vi "Set wavegen SINe signal parameters.vi"(8 "error in (no error)":errorcluster {"code" format="%.0x"}, 9 "Wavegen parameters in":T2={"Frequency (Hz)"=1000.0, "Amplitude (V)"=1.0, "Offset (V)"=0.0, "Load Impedance"=enum."ONEMeg"} {"Offset (V)" format="%#_13g"; "Amplitude (V)" format="%#_13g"; "Frequency (Hz)" min=0.1 max=20000000.0 format="%#_13g"}, 11 "instrument handle in":refnum<k15>) -> (0 "error out":errorcluster, 2 "log string out":string, 3 "instrument handle out":refnum<k15>)   [LabVIEW 2017]
uses:
  Load Impedance.ctl
  Waveform type.ctl
  <instrlib>/Keysight InfiniiVision/Keysight InfiniiVision.lvlib
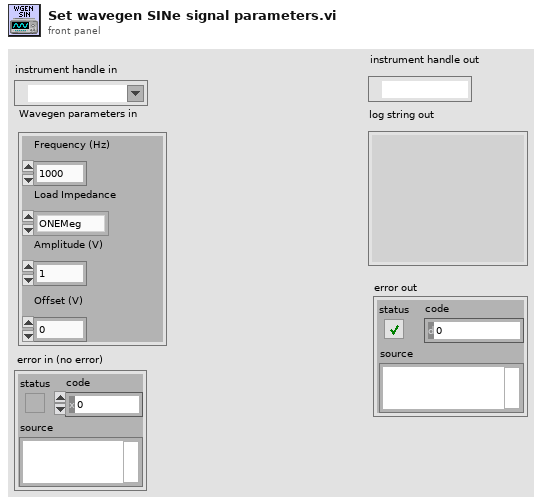
[diagram p1: front panel]
types:
  T1 = typedef "Load Impedance.ctl" = enum16{"ONEMeg", "FIFTy"}
  T2 = cluster{"Frequency (Hz)":dbl, "Amplitude (V)":dbl, "Offset (V)":dbl, "Load Impedance":T1}
  T3 = typedef "Waveform type.ctl" = enum16{"SINe", "SQUare", "RAMP", "PULSe", "DC", "NOISe"}
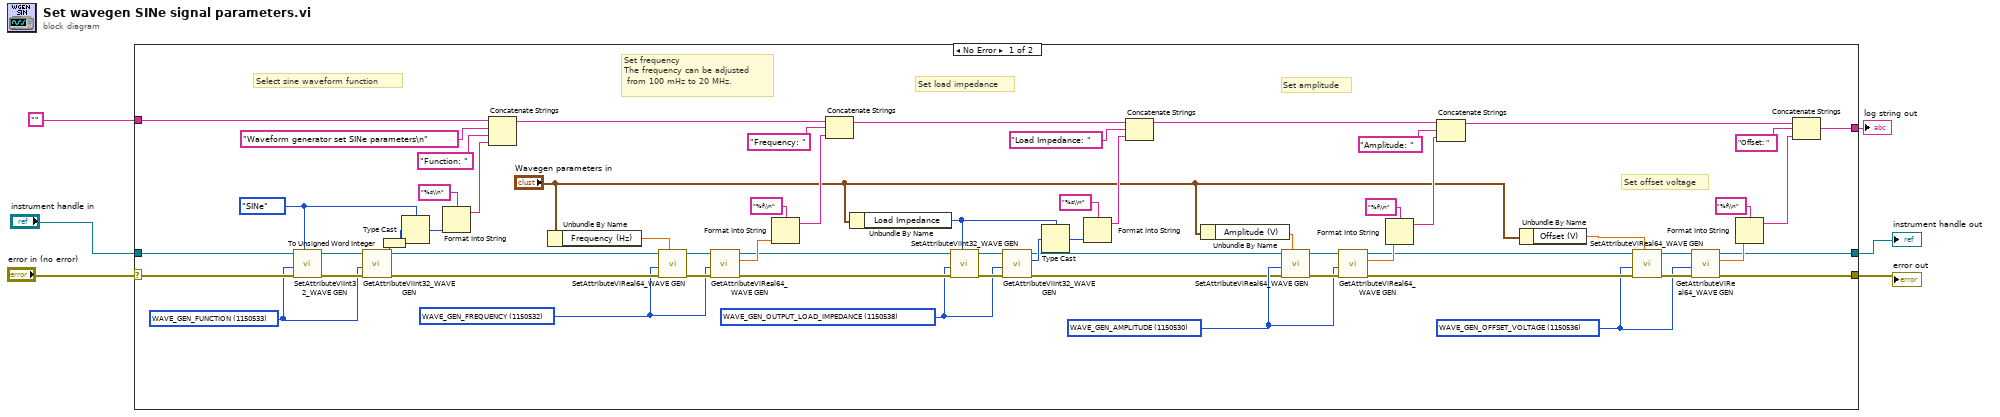
[diagram p0: block diagram]
diagram:
  n1 = case shown="No Error" "error in (no error)" {
    selector: "error in (no error)" -> [w68 w70]
    tunnel: "instrument handle in" -> [w69 w71]
    tunnel: [w34 w71] -> w2
    tunnel: [w33 w70] -> w1
    tunnel: [w32 w72] -> w3
    tunnel: "" ("log string in") -> [w30 w72]
    frame No Error {
      w22 = u32 1150538 items=["ARBITRARY_BYTE_ORDER"=1150415, "MODULATION_FUNCTION"=1150552, "MODULATION_TYPE"=1150555, "TRACKING_PHASE"=1150659, "WAVE_GEN_ADDITIONAL_NOISE"=1150529, "WAVE_GEN_ARBITRARY_BYTE_ORDER"=1150544, "WAVE_GEN_FUNCTION"=1150533, "WAVE_GEN_OUTPUT_LOAD_IMPEDANCE"=1150538, "WAVE_GEN_OUTPUT_MODE"=1150658] ("AttributeID")
      w27 = u32 1150536 items=["FM_DEVIATION"=1150548, "FM_FREQUENCY"=1150549, "FSK_FREQUENCY"=1150550, "FSK_MODULATION_RATE"=1150551, "MODULATION_RAMP_SYMMETRY"=1150553, "WAVE_GEN_AM_DEPTH"=1150546, "WAVE_GEN_AM_FREQUENCY"=1150547, "WAVE_GEN_AMPLITUDE"=1150530, "WAVE_GEN_DUTY_CYCLE"=1150531, "WAVE_GEN_FREQUENCY"=1150532, "WAVE_GEN_HIGH_VOLTAGE"=1150534, "WAVE_GEN_LOW_VOLTAGE"=1150535, "WAVE_GEN_OFFSET_VOLTAGE"=1150536, "WAVE_GEN_PERIOD"=1150539, "WAVE_GEN_PULSE_WIDTH"=1150540, "WAVE_GEN_RAMP_SYMMETRY"=1150541] ("AttributeID")
      w57 = Waveform_type."SINe"
      w28 = u32 1150530 items=["FM_DEVIATION"=1150548, "FM_FREQUENCY"=1150549, "FSK_FREQUENCY"=1150550, "FSK_MODULATION_RATE"=1150551, "MODULATION_RAMP_SYMMETRY"=1150553, "WAVE_GEN_AM_DEPTH"=1150546, "WAVE_GEN_AM_FREQUENCY"=1150547, "WAVE_GEN_AMPLITUDE"=1150530, "WAVE_GEN_DUTY_CYCLE"=1150531, "WAVE_GEN_FREQUENCY"=1150532, "WAVE_GEN_HIGH_VOLTAGE"=1150534, "WAVE_GEN_LOW_VOLTAGE"=1150535, "WAVE_GEN_OFFSET_VOLTAGE"=1150536, "WAVE_GEN_PERIOD"=1150539, "WAVE_GEN_PULSE_WIDTH"=1150540, "WAVE_GEN_RAMP_SYMMETRY"=1150541] ("AttributeID")
      w29 = u32 1150532 items=["FM_DEVIATION"=1150548, "FM_FREQUENCY"=1150549, "FSK_FREQUENCY"=1150550, "FSK_MODULATION_RATE"=1150551, "MODULATION_RAMP_SYMMETRY"=1150553, "WAVE_GEN_AM_DEPTH"=1150546, "WAVE_GEN_AM_FREQUENCY"=1150547, "WAVE_GEN_AMPLITUDE"=1150530, "WAVE_GEN_DUTY_CYCLE"=1150531, "WAVE_GEN_FREQUENCY"=1150532, "WAVE_GEN_HIGH_VOLTAGE"=1150534, "WAVE_GEN_LOW_VOLTAGE"=1150535, "WAVE_GEN_OFFSET_VOLTAGE"=1150536, "WAVE_GEN_PERIOD"=1150539, "WAVE_GEN_PULSE_WIDTH"=1150540, "WAVE_GEN_RAMP_SYMMETRY"=1150541] ("AttributeID")
      w65 = u32 1150533 items=["ARBITRARY_BYTE_ORDER"=1150415, "MODULATION_FUNCTION"=1150552, "MODULATION_TYPE"=1150555, "TRACKING_PHASE"=1150659, "WAVE_GEN_ADDITIONAL_NOISE"=1150529, "WAVE_GEN_ARBITRARY_BYTE_ORDER"=1150544, "WAVE_GEN_FUNCTION"=1150533, "WAVE_GEN_OUTPUT_LOAD_IMPEDANCE"=1150538, "WAVE_GEN_OUTPUT_MODE"=1150658] ("AttributeID")
      # "Set load impedance"
      # "Set offset voltage"
      # "Set amplitude"
      # "Set frequency\nThe frequency can be adjusted\n from 100 mHz to 20 MHz."
      # "Select sine waveform function"
      n2 = call <instrlib>:"SetAttributeViInt32_WAVE GEN.vi"("AttributeValue"=w57, "error in (no error)"=w68, "AttributeID"=w65, "instrument handle"=w69) -> ("error out"=w66:errorcluster, "instrument handle out"=w67:refnum<k15>)  [unwired: 6 in]
      n3 = call <instrlib>:"GetAttributeViInt32_WAVE GEN.vi"("error in (no error)"=w66, "AttributeID"=w65, "instrument handle"=w67) -> ("error out"=w61:errorcluster, "AttributeValue"=w58:i32, "instrument handle out"=w62:refnum<k15>)  [unwired: 6 in]
      n4 = To Unsigned Word Integer(number=w58) -> (unsigned 16bit integer=w7:u16)
      n5 = Type Cast(type=w57, x=w7) -> (*(type *) &x=w56:T3)
      n6 = Format Into String(format string="%s\\n", w56) -> (resulting string=w55:string)  [unwired: 2 in, 1 out]
      n7 = Concatenate Strings(w30, "Waveform generator set SINe parameters\n" ("string"), "Function: " ("string"), w55) -> (w51:string)
      n8 = Unbundle By Name("Wavegen parameters in") -> ("Frequency (Hz)"=w12:dbl)
      n9 = call <instrlib>:"SetAttributeViReal64_WAVE GEN.vi"("AttributeValue"=w12, "error in (no error)"=w61, "AttributeID"=w29, "instrument handle"=w62) -> ("error out"=w63:errorcluster, "instrument handle out"=w64:refnum<k15>)  [unwired: 6 in]
      n10 = call <instrlib>:"GetAttributeViReal64_WAVE GEN.vi"("error in (no error)"=w63, "AttributeID"=w29, "instrument handle"=w64) -> ("error out"=w23:errorcluster, "AttributeValue"=w54:dbl, "instrument handle out"=w24:refnum<k15>)  [unwired: 6 in]
      n11 = Format Into String(format string="%f\\n", w54) -> (resulting string=w49:string)  [unwired: 2 in, 1 out]
      n12 = Concatenate Strings(w51, "Frequency: " ("string"), w49) -> (w17:string)
      n13 = Unbundle By Name("Wavegen parameters in") -> ("Load Impedance"=w11:T1)
      n14 = call <instrlib>:"SetAttributeViInt32_WAVE GEN.vi"("AttributeValue"=w11, "error in (no error)"=w23, "AttributeID"=w22, "instrument handle"=w24) -> ("error out"=w26:errorcluster, "instrument handle out"=w25:refnum<k15>)  [unwired: 6 in]
      n15 = call <instrlib>:"GetAttributeViInt32_WAVE GEN.vi"("error in (no error)"=w26, "AttributeID"=w22, "instrument handle"=w25) -> ("error out"=w14:errorcluster, "AttributeValue"=w19:i32, "instrument handle out"=w13:refnum<k15>)  [unwired: 6 in]
      n16 = Type Cast(type=w11, x=w19) -> (*(type *) &x=w21:T1)
      n17 = Format Into String(format string="%s\\n", w21) -> (resulting string=w16:string)  [unwired: 2 in, 1 out]
      n18 = Concatenate Strings(w17, "Load Impedance: " ("string"), w16) -> (w15:string)
      n19 = Unbundle By Name("Wavegen parameters in") -> ("Amplitude (V)"=w10:dbl)
      n20 = call <instrlib>:"SetAttributeViReal64_WAVE GEN.vi"("AttributeValue"=w10, "error in (no error)"=w14, "AttributeID"=w28, "instrument handle"=w13) -> ("error out"=w59:errorcluster, "instrument handle out"=w60:refnum<k15>)  [unwired: 6 in]
      n21 = call <instrlib>:"GetAttributeViReal64_WAVE GEN.vi"("error in (no error)"=w59, "AttributeID"=w28, "instrument handle"=w60) -> ("error out"=w37:errorcluster, "AttributeValue"=w39:dbl, "instrument handle out"=w38:refnum<k15>)  [unwired: 6 in]
      n22 = Format Into String(format string="%f\\n", w39) -> (resulting string=w45:string)  [unwired: 2 in, 1 out]
      n23 = Concatenate Strings(w15, "Amplitude: " ("string"), w45) -> (w35:string)
      n24 = Unbundle By Name("Wavegen parameters in") -> ("Offset (V)"=w9:dbl)
      n25 = call <instrlib>:"SetAttributeViReal64_WAVE GEN.vi"("AttributeValue"=w9, "error in (no error)"=w37, "AttributeID"=w27, "instrument handle"=w38) -> ("error out"=w43:errorcluster, "instrument handle out"=w44:refnum<k15>)  [unwired: 6 in]
      n26 = call <instrlib>:"GetAttributeViReal64_WAVE GEN.vi"("error in (no error)"=w43, "AttributeID"=w27, "instrument handle"=w44) -> ("error out"=w33:errorcluster, "AttributeValue"=w36:dbl, "instrument handle out"=w34:refnum<k15>)  [unwired: 6 in]
      n27 = Format Into String(format string="%f\\n", w36) -> (resulting string=w40:string)  [unwired: 2 in, 1 out]
      n28 = Concatenate Strings(w35, "Offset: " ("string"), w40) -> (w32:string)
    }
    frame Error {
    }
  }
  "log string out" <- w3
  "instrument handle out" <- w2
  "error out" <- w1
